vi "Configure Composite Limit Test.vi"(8 "error in (no error)":errorcluster, 9 "4-bit Pass Pattern (1111)":i32=15 min=0 max=15 format="%b", 10 "Enable Auto Clear (F)":bool, 11 "VISA resource name":refnum<visa-resource-name>) -> (0 "error out":errorcluster, 3 "VISA resource name out":refnum<visa-resource-name>)   [LabVIEW 2019, in "Keithley 6517.lvlib"]
doc: "Configures the Composite Limit test.\n\n<B>Note:</B>\nThis VI is ONLY compatible with <B>model 6514</B>. Running this VI with any other model will result in an error."
uses:
  Keithley 6517.lvlib
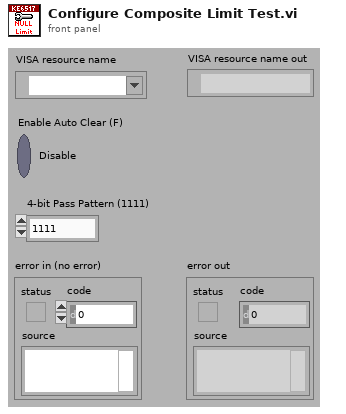
[diagram p1: front panel]
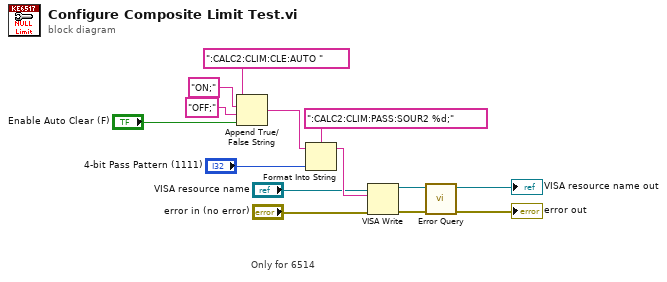
[diagram p0: block diagram]
diagram:
  # "Only for 6514"
  n1 = Append True/False String(1:"Enable Auto Clear (F)", 2:"OFF;" ("false string"), 3:"ON;" ("true string"), 4:":CALC2:CLIM:CLE:AUTO " ("command")) -> (0:w8:string)
  n2 = Format Into String(format string=":CALC2:CLIM:PASS:SOUR2 %d;", initial string=w8, "4-bit Pass Pattern (1111)") -> (resulting string=w3:string)  [unwired: 1 in, 1 out]
  n3 = VISA Write(VISA resource name="VISA resource name", write buffer=w3, error in (no error)="error in (no error)") -> (VISA resource name out=w6:refnum<visa-resource-name>, error out=w7:errorcluster)  [unwired: 1 out]
  n4 = call "Error Query.vi"("error in (no error)"=w7, "VISA resource name"=w6) -> ("error out"=→"error out":errorcluster, "VISA resource name out"=→"VISA resource name out":refnum<visa-resource-name>)  [unwired: 6 in, 2 out]
